vi "MVS.vi"(0 "System no.":i32=1 min=1 step=1, 2 "Axes to move":string[](array[string]), 3 "Position values":dbl[](array[numeric]) format="%.6f", 4 "No.of digits\nfor Pos. values":i16=4, 5 "error in":errorcluster, 6 "Step size":dbl[](array[numeric]) format="%.6f", 7 "No.of digits\nfor Step size":i16=4, 8 "Delay time (ms)":dbl[](array[numeric])) -> (19 "error out":errorcluster)   [LabVIEW 2020]
doc: "MoVe given axes in Steps relative to their current position. The new target position is calculated by adding \"Position values\" to the last commanded target values. The movement is performed in steps with the size of \"Step size\". After each step a delay of \"Delay time (ms)\" (in milliseconds) takes place.\nDuring the execution of the command, the controller is in \"not ready\" state, which can be checked by the #7 command.\nThis command can be interrupted by #24, HLT and STP.\nServo must be enabled prior to using this command.\nNote: The Step size is automatically adapted so that the resulting number of steps is an integer value. \nNo. of digits is the number of digits after the decimal point in the position and step size value(s) that will be sent."
panel:
  # "MoVe given axes in Steps relative to their current position."
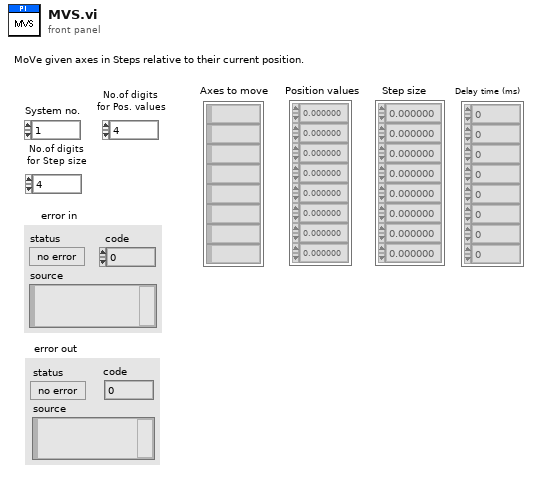
[diagram p1: front panel]
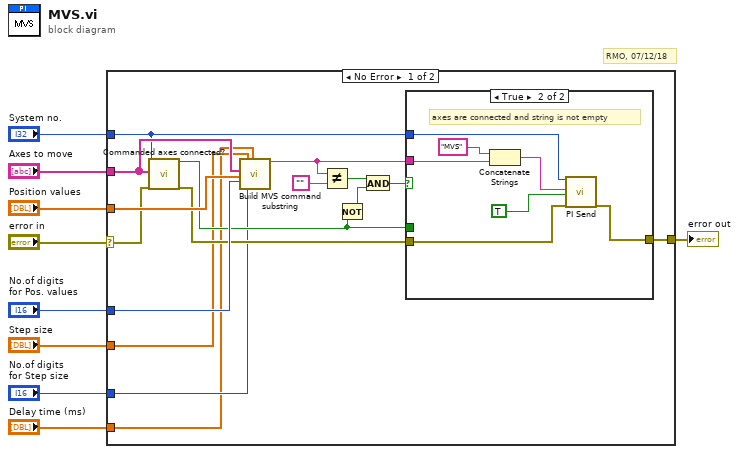
[diagram p0: block diagram]
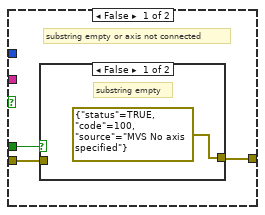
[diagram p2: hidden frame]
diagram:
  # "RMO, 07/12/18"
  n1 = case shown="No Error" "error in" {
    selector: "error in" -> [w10 w38]
    tunnel: [w25 w38] -> w9
    tunnel: "Position values" -> [w22 _]
    tunnel: "No.of digits\nfor Pos. values" -> [w21 _]
    tunnel: "System no." -> [w14 _]
    tunnel: "Axes to move" -> [w19 _]
    tunnel: "Step size" -> [w13 _]
    tunnel: "No.of digits\nfor Step size" -> [w12 _]
    tunnel: "Delay time (ms)" -> [w11 _]
    frame No Error {
      n2 = call "Commanded axes connected?.vi"("System no."=w14, "Commanded axes"=w19, "error in"=w10) -> ("Controller error"=w17:bool, "error out"=w20:errorcluster)  [unwired: 1 in, 14 out]
      n3 = call "Build MVS command substring.vi"("Affected axes"=w19, "Position values"=w22, "No.of digits\nfor Pos. values"=w21, "Step size"=w13, "No.of digits\nfor Step size"=w12, "Delay time"=w11) -> ("Command substring"=w23:string)  [unwired: 1 in, 12 out]
      n4 = Not Equal?(x=w23, y="") -> (x != y?=w18:bool)
      n5 = Not(x=w17) -> (.not. x?=w16:bool)
      n6 = And(x=w18, y=w16) -> (x .and. y?=w15:bool)
      n7 = case shown="True" w15 {
        tunnel: w23 -> [_ w36]
        tunnel: [w28 w32] -> w25
        tunnel: w20 -> [w26 w33]
        tunnel: w17 -> [w27 _]
        tunnel: w14 -> [_ w31]
        frame False {
          # "substring empty or axis not connected"
          n8 = case shown="False" w27 {
            tunnel: [errorcluster {"status"=TRUE, "code"=100, "source"="MVS No axis specified"} ("error out") w30] -> w28
            tunnel: w26 -> [_ w30]
            frame False {
              # "substring empty"
            }
            frame True {
              # "commanded axis not connected"
            }
          }
        }
        frame True {
          # "axes are connected and string is not empty"
          n9 = Concatenate Strings("MVS", w36) -> (w34:string)
          n10 = call "PI Send.vi"("System no."=w31, "String to send"=w34, "Attach termination char.?"=TRUE ("Attach Linefeed?"), "error in"=w33) -> ("error out"=w32:errorcluster)  [unwired: 2 in, 13 out]
        }
      }
    }
    frame Error {
    }
  }
  "error out" <- w9
